vi "Get Pars Labels.vi"(11 "Spectral Data In":T1={"PDT Amp [v]"=0.0, "RIS Amp [v]"=0.0, "B-Field"=[], "All In-Phase Scan Spectra"=[], "Model Select"=enum."OneCompRISTwoPDT", "Fit Each Scan"=FALSE, "PDT Center [g]"=0.0, "In-Phase Average Spectra"=[], "In-Phase Median Spectra"=[], "Out-Phase Median Spectra"=[], "Out-Phase Average Spectra"=[], "Fit Spectra"=[], "Fit No-Baseline Spectra"=[], "All Out-Phase Scan Spectra"=[], "Baseline Offset Correction"=FALSE, "In-Phase Offset [v]"=0.0, "Out-Phase Offset [v]"=0.0, "Ch2 Input\n(Balance)"=[], "Ch3 Input\n(Phase)"=[], "Ch4 Input\n(AFC)"=[], "Fit Pars"=[], "Fit Pars Errors"=[], "Fit Pars Labels"=[], "Raw Scan DAQ Data"=[], "Bad Scans Indicies"=[], "Good In-Phase Scan Spectra"=[], "Good Out-Phase Scan Spectra"=[], "Bad In-Phase Scan Spectra"=[], "Bad Out-Phase Scan Spectra"=[], "Number of bad scans"=0, "Fit History"=[], "PDT Amp. History/Set [v]"=[], "RIS Amp. History/Set [v]"=[], "RIS Amp. History/Scan [v]"=[], "All Shifted B-Fields"=[], "Good Shifted B-Fields"=[], "Ch5 Input\n(SpO2)"=[], "Ch6 Input\n(BPM)"=[], "Global SNR"=0.0, "Fit Error History"=[], "SNR History"=[]} {"Global SNR" min=0.0; "PDT Center [g]" min=0.0; "RIS Amp [v]" min=0.0}) -> (3 "Pars Labels":string[](array[string]))   [LabVIEW 2016]
uses:
  EPR DAQ/qsm/trunk/Types/Spectral Data.ctl
  EPR DAQ/qsm/trunk/Types/Fitting Model Selection.ctl
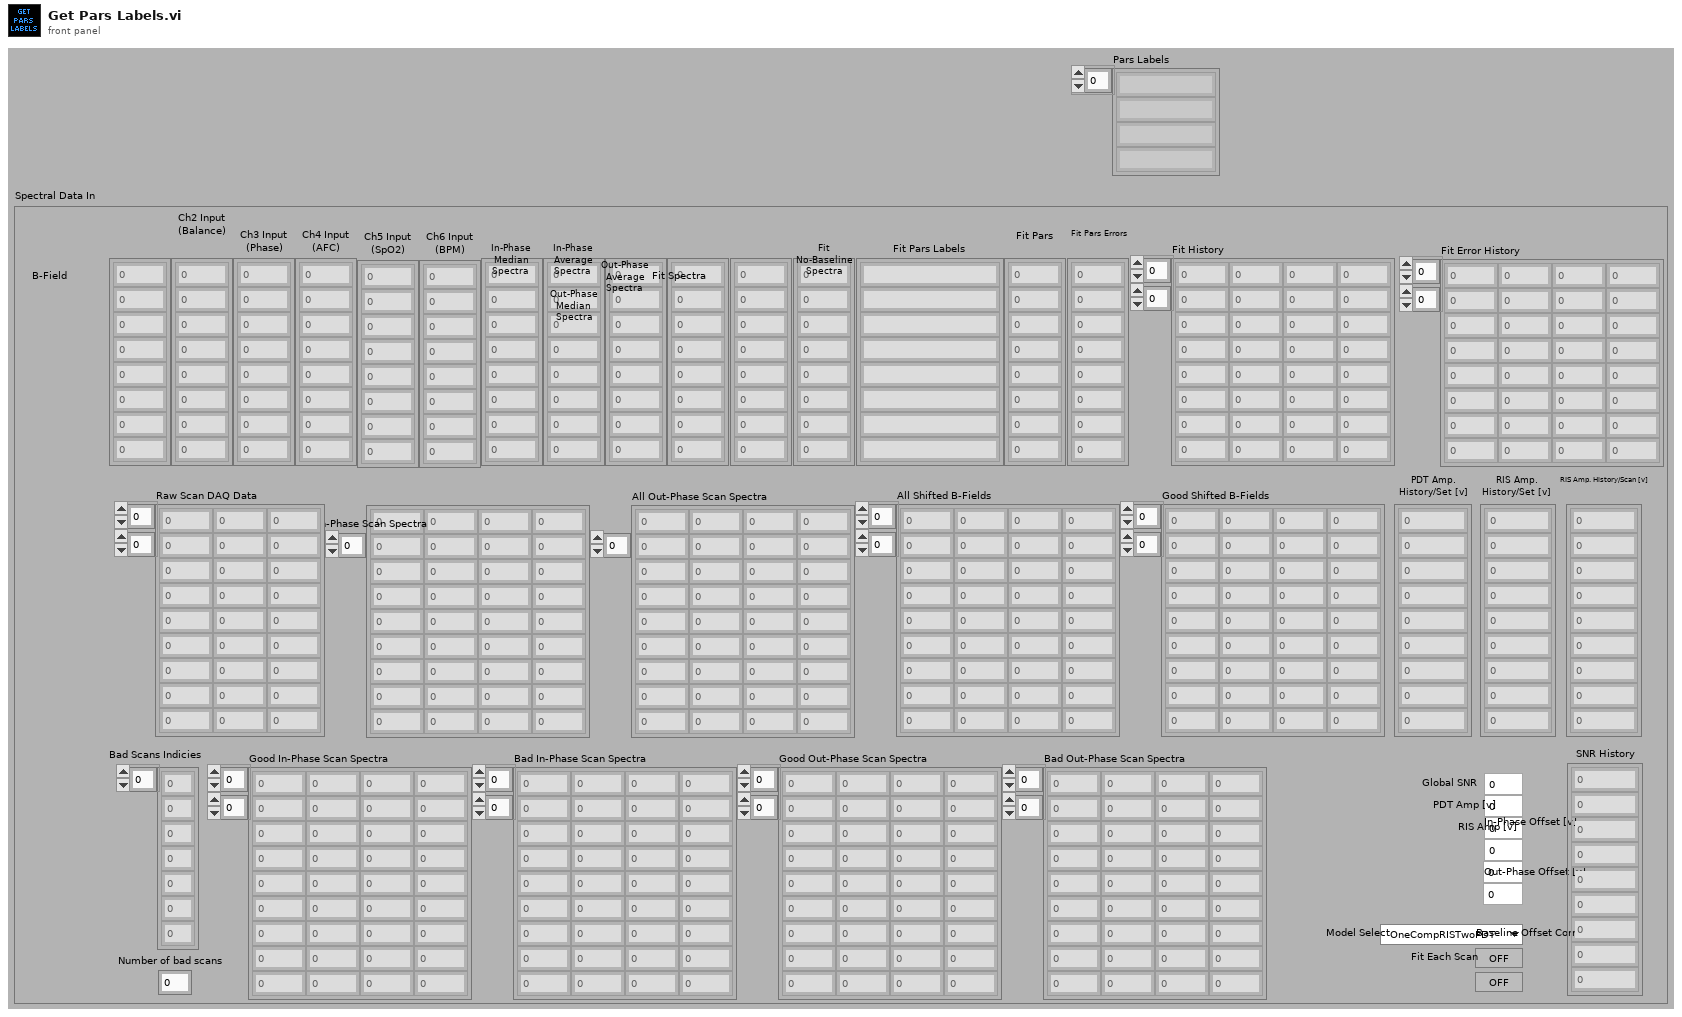
[diagram p1: front panel]
types:
  T1 = typedef "Spectral Data.ctl" = cluster{"PDT Amp [v]":dbl, "RIS Amp [v]":dbl, "B-Field":dbl[], "All In-Phase Scan Spectra":dbl[][], "Model Select":T2, "Fit Each Scan":bool, "PDT Center [g]":dbl, "In-Phase Average Spectra":dbl[], "In-Phase Median Spectra":dbl[], "Out-Phase Median Spectra":dbl[], "Out-Phase Average Spectra":dbl[], "Fit Spectra":dbl[], "Fit No-Baseline Spectra":dbl[], "All Out-Phase Scan Spectra":dbl[][], "Baseline Offset Correction":bool, "In-Phase Offset [v]":dbl, "Out-Phase Offset [v]":dbl, "Ch2 Input\n(Balance)":dbl[], "Ch3 Input\n(Phase)":dbl[], "Ch4 Input\n(AFC)":dbl[], "Fit Pars":dbl[], "Fit Pars Errors":dbl[], "Fit Pars Labels":string[], "Raw Scan DAQ Data":dbl[][], "Bad Scans Indicies":i32[], "Good In-Phase Scan Spectra":dbl[][], "Good Out-Phase Scan Spectra":dbl[][], "Bad In-Phase Scan Spectra":dbl[][], "Bad Out-Phase Scan Spectra":dbl[][], "Number of bad scans":i32, "Fit History":dbl[][], "PDT Amp. History/Set [v]":dbl[], "RIS Amp. History/Set [v]":dbl[], "RIS Amp. History/Scan [v]":dbl[], "All Shifted B-Fields":dbl[][], "Good Shifted B-Fields":dbl[][], "Ch5 Input\n(SpO2)":dbl[], "Ch6 Input\n(BPM)":dbl[], "Global SNR":dbl, "Fit Error History":dbl[][], "SNR History":dbl[]}
  T2 = typedef "Fitting Model Selection.ctl" = enum16{"OneCompRIS", "OneCompRISTwoPDT", "OneCompRISRev", "OneCompRISTwoPDTRev", "LiPc", "TwoLiPc", "ThreeLiPc", "FourLiPc", "PDTCalibration", "CE_Ink", "Printex", "MelaninTwoPDT"}
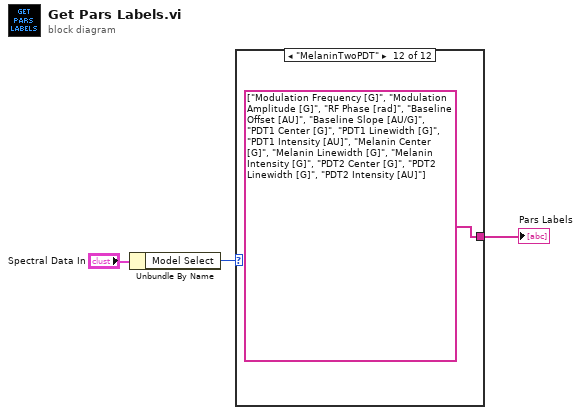
[diagram p0: block diagram]
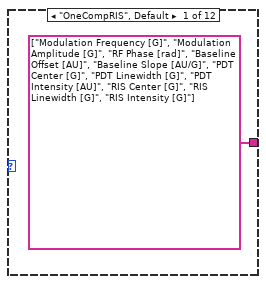
[diagram p2: hidden frame]
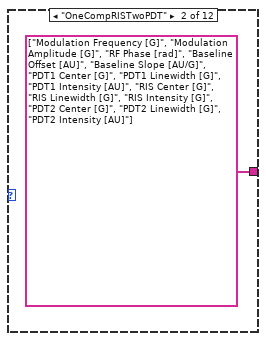
[diagram p3: hidden frame]
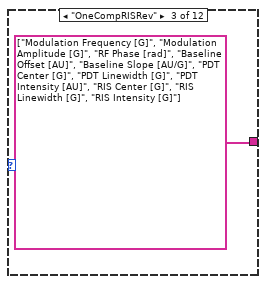
[diagram p4: hidden frame]
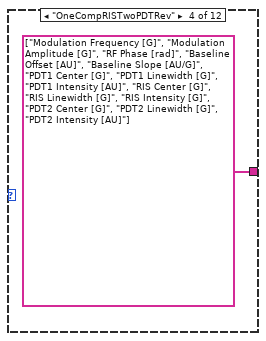
[diagram p5: hidden frame]
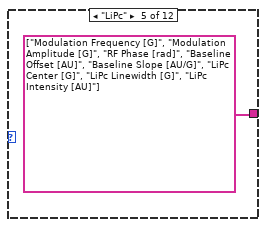
[diagram p6: hidden frame]
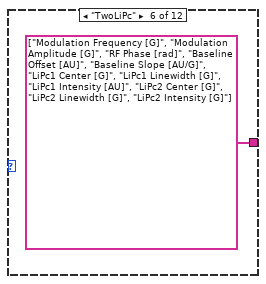
[diagram p7: hidden frame]
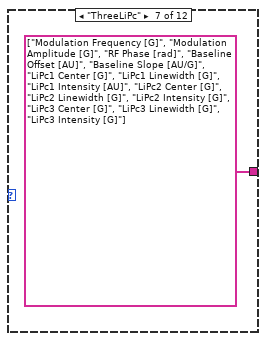
[diagram p8: hidden frame]
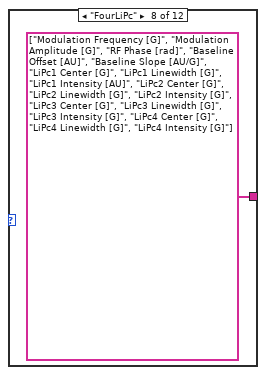
[diagram p9: hidden frame]
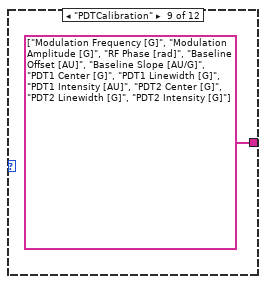
[diagram p10: hidden frame]
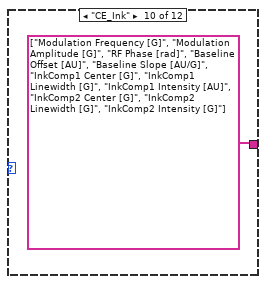
[diagram p11: hidden frame]
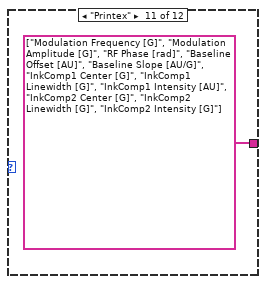
[diagram p12: hidden frame]
diagram:
  n1 = Unbundle By Name("Spectral Data In") -> ("Model Select"=w2:T2)
  n2 = case shown="\"MelaninTwoPDT\"" w2 {
    tunnel: [string[] ["Modulation Frequency [G]", "Modulation Amplitude [G]", "RF Phase [rad]", "Baseline Offset [AU]", "Baseline Slope [AU/G]", "PDT Center [G]", "PDT Linewidth [G]", "PDT Intensity [AU]", "RIS Center [G]", "RIS Linewidth [G]", "RIS Intensity [G]"] string[] ["Modulation Frequency [G]", "Modulation Amplitude [G]", "RF Phase [rad]", "Baseline Offset [AU]", "Baseline Slope [AU/G]", "PDT1 Center [G]", "PDT1 Linewidth [G]", "PDT1 Intensity [AU]", "RIS Center [G]", "RIS Linewidth [G]", "RIS Intensity [G]", "PDT2 Center [G]", "PDT2 Linewidth [G]", "PDT2 Intensity [AU]"] string[] ["Modulation Frequency [G]", "Modulation Amplitude [G]", "RF Phase [rad]", "Baseline Offset [AU]", "Baseline Slope [AU/G]", "PDT Center [G]", "PDT Linewidth [G]", "PDT Intensity [AU]", "RIS Center [G]", "RIS Linewidth [G]", "RIS Intensity [G]"] string[] ["Modulation Frequency [G]", "Modulation Amplitude [G]", "RF Phase [rad]", "Baseline Offset [AU]", "Baseline Slope [AU/G]", "PDT1 Center [G]", "PDT1 Linewidth [G]", "PDT1 Intensity [AU]", "RIS Center [G]", "RIS Linewidth [G]", "RIS Intensity [G]", "PDT2 Center [G]", "PDT2 Linewidth [G]", "PDT2 Intensity [AU]"] string[] ["Modulation Frequency [G]", "Modulation Amplitude [G]", "RF Phase [rad]", "Baseline Offset [AU]", "Baseline Slope [AU/G]", "LiPc Center [G]", "LiPc Linewidth [G]", "LiPc Intensity [AU]"] string[] ["Modulation Frequency [G]", "Modulation Amplitude [G]", "RF Phase [rad]", "Baseline Offset [AU]", "Baseline Slope [AU/G]", "LiPc1 Center [G]", "LiPc1 Linewidth [G]", "LiPc1 Intensity [AU]", "LiPc2 Center [G]", "LiPc2 Linewidth [G]", "LiPc2 Intensity [G]"] string[] ["Modulation Frequency [G]", "Modulation Amplitude [G]", "RF Phase [rad]", "Baseline Offset [AU]", "Baseline Slope [AU/G]", "LiPc1 Center [G]", "LiPc1 Linewidth [G]", "LiPc1 Intensity [AU]", "LiPc2 Center [G]", "LiPc2 Linewidth [G]", "LiPc2 Intensity [G]", "LiPc3 Center [G]", "LiPc3 Linewidth [G]", "LiPc3 Intensity [G]"] string[] ["Modulation Frequency [G]", "Modulation Amplitude [G]", "RF Phase [rad]", "Baseline Offset [AU]", "Baseline Slope [AU/G]", "LiPc1 Center [G]", "LiPc1 Linewidth [G]", "LiPc1 Intensity [AU]", "LiPc2 Center [G]", "LiPc2 Linewidth [G]", "LiPc2 Intensity [G]", "LiPc3 Center [G]", "LiPc3 Linewidth [G]", "LiPc3 Intensity [G]", "LiPc4 Center [G]", "LiPc4 Linewidth [G]", "LiPc4 Intensity [G]"] string[] ["Modulation Frequency [G]", "Modulation Amplitude [G]", "RF Phase [rad]", "Baseline Offset [AU]", "Baseline Slope [AU/G]", "PDT1 Center [G]", "PDT1 Linewidth [G]", "PDT1 Intensity [AU]", "PDT2 Center [G]", "PDT2 Linewidth [G]", "PDT2 Intensity [G]"] string[] ["Modulation Frequency [G]", "Modulation Amplitude [G]", "RF Phase [rad]", "Baseline Offset [AU]", "Baseline Slope [AU/G]", "InkComp1 Center [G]", "InkComp1 Linewidth [G]", "InkComp1 Intensity [AU]", "InkComp2 Center [G]", "InkComp2 Linewidth [G]", "InkComp2 Intensity [G]"] string[] ["Modulation Frequency [G]", "Modulation Amplitude [G]", "RF Phase [rad]", "Baseline Offset [AU]", "Baseline Slope [AU/G]", "InkComp1 Center [G]", "InkComp1 Linewidth [G]", "InkComp1 Intensity [AU]", "InkComp2 Center [G]", "InkComp2 Linewidth [G]", "InkComp2 Intensity [G]"] string[] ["Modulation Frequency [G]", "Modulation Amplitude [G]", "RF Phase [rad]", "Baseline Offset [AU]", "Baseline Slope [AU/G]", "PDT1 Center [G]", "PDT1 Linewidth [G]", "PDT1 Intensity [AU]", "Melanin Center [G]", "Melanin Linewidth [G]", "Melanin Intensity [G]", "PDT2 Center [G]", "PDT2 Linewidth [G]", "PDT2 Intensity [AU]"]] -> w1
    frame "OneCompRIS", Default {
    }
    frame "OneCompRISTwoPDT" {
    }
    frame "OneCompRISRev" {
    }
    frame "OneCompRISTwoPDTRev" {
    }
    frame "LiPc" {
    }
    frame "TwoLiPc" {
    }
    frame "ThreeLiPc" {
    }
    frame "FourLiPc" {
    }
    frame "PDTCalibration" {
    }
    frame "CE_Ink" {
    }
    frame "Printex" {
    }
    frame "MelaninTwoPDT" {
    }
  }
  "Pars Labels" <- w1
